vi "Analyze Coefficients-Quantized Multistage Multirate Filter.vi"() -> ()   [LabVIEW 2023]
doc: "Demonstrates how to use the DFD FXP NStage MRate Quantization VI to quantize the coefficients of a floating-point multistage multirate filter and use the DFD Plot NStage MRate Freq Response VI to analyze a quantized multistage multirate filter.\n\nComplete the following steps to use this VI.\n1) Run the VI. This VI first designs a floating-point multistage multirate filter using pre-defined values and then quantizes the multirate filter coefficients.\n2) Observe the Magnitude Responses graph. This graph displays the magnitude responses of both the fixed-point multirate filter and the reference floating-point multirate filter.\n3) From the <B>Stage View</B> pull-down menu, select each item to view the magnitude responses of the corresponding stage.\n4) Modify the <B>Coefficients Word Lengths</B> and <B>Scale Type</B> settings and see how your changes affect the magnitude responses.\n5) Click the <B>STOP</B> button to stop this VI.\n6) Examine the block diagram of this VI to obtain information about using the DFD FXP NStage MRate Quantization VI and the DFD Plot NStage MRate Freq Response VI."
uses:
  <vilib>/addons/Digital Filter Design/_Objects.llb/DFD Coef Norm Type.ctl
  <vilib>/addons/Digital Filter Design/_Objects.llb/DFD Multirate Filtering Mode.ctl
  <vilib>/addons/Digital Filter Design/_Objects.llb/DFD Filter Ripple Specification (Design).ctl
  <vilib>/addons/Digital Filter Design/_Objects.llb/DFD Multirate Filter Specification (Design).ctl
  <vilib>/addons/Digital Filter Design/NI_DigFilterLicensed.lvlib
panel:
  in  "stop":bool
  in  "Stage View":u16(ring) items=["Overall", "Stage 1", "Stage 2"]
  in  "Scale by Power of 2?":bool
  in  "Scale Type":T1=enum."Time Domain 1-Norm"
  in  "Coefficients Word Lengths":i16[](array[numeric])=[16, 16]
  out "Error Message":string
  out "Magnitude Responses":cluster{"f0":dbl, "df":dbl, "values":dbl[]}[](graph)
  # "Select Help>>Show Context Help and move the cursor over the VI icon for more information."
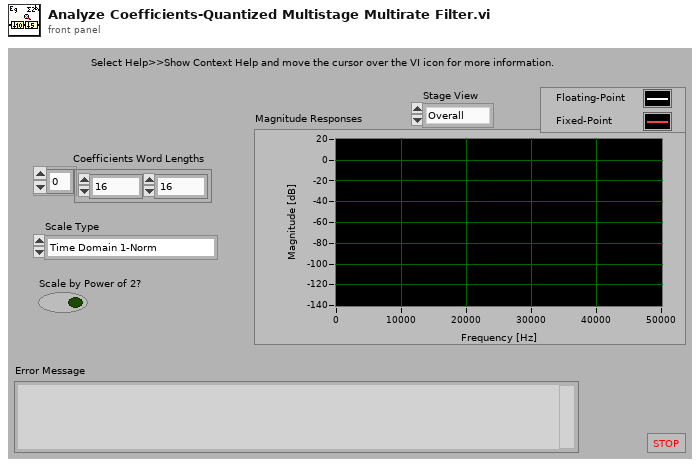
[diagram p1: front panel]
types:
  T1 = typedef "NI_DigFilterLicensed.lvlib/DFD Coef Norm Type.ctl" = enum16{"No Norm", "Time Domain 1-Norm", "Time Domain 2-Norm", "Time Domain Inf-Norm"}
  T2 = typedef "NI_DigFilterLicensed.lvlib/DFD Multirate Filter Specification (Design).ctl" = cluster{"fpass":dbl, "fstop":dbl}
  T3 = typedef "NI_DigFilterLicensed.lvlib/DFD Filter Ripple Specification (Design).ctl" = cluster{"passband":dbl, "stopband":dbl, "dB/linear? (T: dB)":bool}
  T4 = typedef "NI_DigFilterLicensed.lvlib/DFD Multirate Filtering Mode.ctl" = u16
  T5 = typedef "NI_DigFilterLicensed.lvlib/DFD Multirate Filter Obj.ctl" = cluster{"mMRate_Structure":enum16{"CIC", "FIR", "IIR", "Lattice"}, "mMRate_Mode":T6, "mMRate_Factor":i32, "mMRate_FIRParams":cluster{"mMRate_FIR_H":dbl[], "mMRate_FIR_IsNyquist?":bool, "mMRate_FIR_IsSymmetric?":bool}, "mMRate_CICParams":cluster{"mMRate_CIC_#Stage":i32, "mMRate_CIC_Lag":i32, "mMRate_CIC_Type":enum16{"Lowpass", "Highpass"}}, "mMRate_Order":i32, "mMRate_Version":string, "mMRate_Comments":string, "mMRate_RationalFactor":cluster{"mMRate_L":i32, "mMRate_M":i32}, "mMRate_Fs":dbl, "mMRate_Quantized?":bool, "mMRate_QFilterGain":dbl, "mMRate_CoefWl":i16, "mMRate_Scaling":cluster{"mMRate_ScaleByPowerOf2?":bool, "mMRate_ScaleType":T1}, "mMRate_InputWl":i16, "mMRate_OutputWl":i16, "mMRate_OutputMode":T7, "mMRate_MultMode":T8, "mMRate_BitPruning":bool, "mMRate_GainWl":i16, "mMRate_OutputFwl":i16, "mMRate_SumIwl":i16, "mMRate_InputIwl ":i16, "mMRate_SumWl":i16, "mMRate_CoefIwl":i16}
  T6 = typedef "NI_DigFilterLicensed.lvlib/DFD Multirate Mode.ctl" = i16
  T7 = typedef "NI_DigFilterLicensed.lvlib/DFD Round-off Mode.ctl" = enum16{"Nearest", "Truncation"}
  T8 = typedef "NI_DigFilterLicensed.lvlib/DFD FXP MRate Multiply Mode.ctl" = enum16{"Truncated", "Full"}
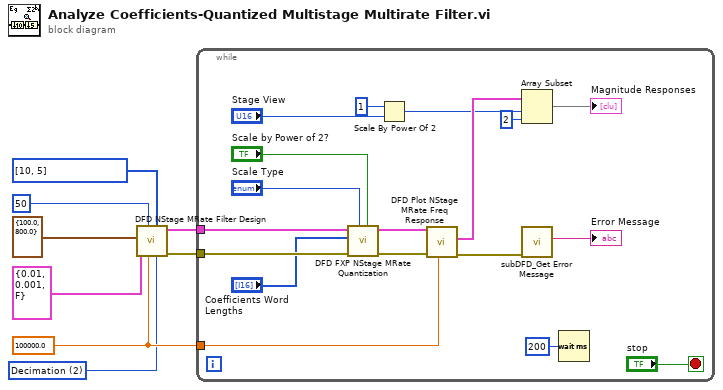
[diagram p0: block diagram]
diagram:
  w3 = 100000.0 ("Sampling Rate [Hz]")
  w2 = T4 2 items=["No Rate Change", "Interpolation", "Decimation"] ("Filtering Mode")
  n1 = call <vilib>:"DFD NStage MRate Filter Design.vi"("filtering mode"=w2, "manual factorization"=i32[] [10, 5] ("Manual Factorization"), "fs in [Hz]"=w3, "factor"=50 ("Factor"), "ripple specs"=T3 {"passband"=0.01, "stopband"=0.001, "dB/linear? (T: dB)"=FALSE} ("Ripple Specs"), "freq specs [Hz]"=T2 {"fpass"=100.0, "fstop"=800.0} ("Freq Spec")) -> ("error out"=w1:errorcluster, "multirate filters out"=w6:T5[])  [unwired: 2 in, 2 out]
  n2 = while {
    tunnel: w6 -> [w26]
    tunnel: w3 -> [w24]
    tunnel: w1 -> [w20]
    stop <- "stop" stop-if-true
    n3 = call <vilib>:"DFD FXP NStage MRate Quantization.vi"("scale by power of 2? (F)"="Scale by Power of 2?", "scale type"="Scale Type", "error in (no error)"=w20, "coefficients word lengths"="Coefficients Word Lengths", "multirate filters in"=w26) -> ("error out"=w19:errorcluster, "multirate filters out"=w21:T5[])  [unwired: 1 in, 4 out]
    n4 = Scale By Power Of 2(n=1, x="Stage View") -> (x*2^n=w12:u16)
    n5 = call <vilib>:"DFD Plot NStage MRate Freq Response.vi"("fs in [Hz]"=w24, "error in (no error)"=w19, "multirate filters in"=w21) -> ("error out"=w22:errorcluster, "magnitude responses"=w25:cluster{"f0":dbl, "df":dbl, "values":dbl[]}[])  [unwired: 4 in, 3 out]
    n6 = Array Subset(array=w25, index=w12, length=2) -> (→"Magnitude Responses":cluster{"f0":dbl, "df":dbl, "values":dbl[]}[])
    n7 = call <vilib>:"subDFD_Get Error Message.vi"("error in (no error)"=w22) -> ("Error Message"=→"Error Message":string)  [unwired: 10 out]
    n8 = Wait (ms)(milliseconds to wait=u32 200) -> ()  [unwired: 1 out]
  }
